vi "Set Attenuation, 400 MHz Power, and 2.45 GHz Power.vi"(6 "2.45 GHz Wake-Up Power (6)":i8(ring)=6 items=["-29"=-29, "-4"=-4, "-2"=-2, "0"=0, "2"=2, "4"=4, "6"=6, "8"=8, "10"=10, "12"=12, "14"=14, "16"=16, "18"=18, "20"=20, "22"=22, "24"=24, "26"=26, "27"=27], 8 "error in":errorcluster, 9 "Attenuation dB (0)":dbl, 10 "400 MHz MICS Power Setting (0x16)":u8=22 format="%.0x", 11 "VISA Resource Name":refnum<visa-resource-name>) -> (0 "error out":errorcluster, 3 "dup VISA Resource Name":refnum<visa-resource-name>)   [LabVIEW 2020]
uses:
  MICS Parameters Global.vi
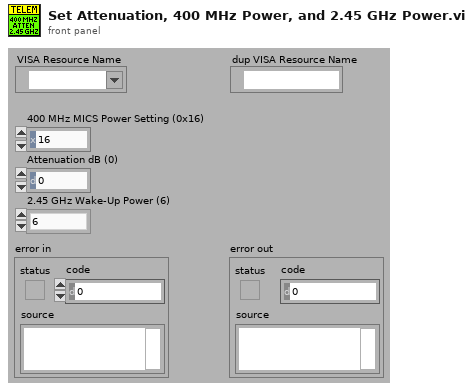
[diagram p1: front panel]
types:
  T1 = cluster{"ConfigFlags":u8, "ImplantID":u32, "CompanyID":u8, "Normal_Comm":cluster{"RF_Channel":u8, "UserData":u8, "TX_Mod":u8, "RX_Mod":u8, "RX_BlockSize":u8, "BlockPerPack":u8, "TX_BlockSize":u8}, "Emerg_Comm":cluster{"RF_Channel":u8, "UserData":u8, "TX_Mod":u8, "RX_Mod":u8, "TX_BlockSize":u8, "BlockPerPack":u8, "RX_BlockSize":u8}, "ImplantRev":u8, "245TX_PowerCal":i8, "245TX_Power":i8, "CCA_RSSI_Thresholds":cluster{"ch0":u16, "ch1":u16, "ch2":u16, "ch3":u16, "ch4":u16, "ch5":u16, "ch6":u16, "ch7":u16, "ch8":u16, "ch9":u16}}
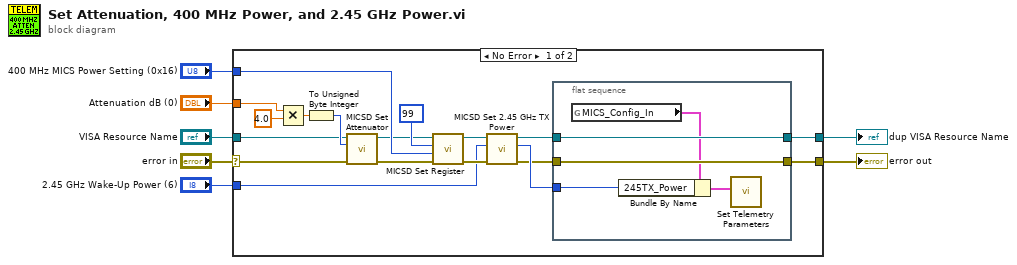
[diagram p0: block diagram]
diagram:
  n1 = case shown="No Error" "error in" {
    selector: "error in" -> [w12 w31]
    tunnel: "400 MHz MICS Power Setting (0x16)" -> [w25 _]
    tunnel: "Attenuation dB (0)" -> [w20 _]
    tunnel: "VISA Resource Name" -> [w17 w32]
    tunnel: [w10 w32] -> w4
    tunnel: [w8 w31] -> w3
    tunnel: "2.45 GHz Wake-Up Power (6)" -> [w13 _]
    frame No Error {
      n2 = Multiply(x=w20, y=4.0) -> (x*y=w18:dbl)
      n3 = To Unsigned Byte Integer(number=w18) -> (unsigned 8bit integer=w21:u8)
      n4 = call "MICSD Set Attenuator.vi"("error in (no error)"=w12, "Attenuation"=w21, "VISA Resource Name"=w17) -> ("error out"=w23:errorcluster, "dup VISA Resource Name"=w22:refnum<visa-resource-name>)  [unwired: 7 in]
      n5 = call "MICSD Set Register.vi"("error in (no error)"=w23, "Data"=w25, "Address"=u16 99, "VISA Resource Name"=w22) -> ("error out"=w15:errorcluster, "dup VISA Resource Name"=w16:refnum<visa-resource-name>)  [unwired: 6 in]
      n6 = call "MICSD Set 2.45 GHz TX Power.vi"("error in (no error)"=w15, "245TX_Power"=w13, "VISA Resource Name"=w16) -> ("error out"=w9:errorcluster, "dup 245TX_Power"=w14:i8, "dup VISA Resource Name"=w11:refnum<visa-resource-name>)  [unwired: 6 in]
      n7 = flat-sequence {
        tunnel: w14 -> [w30]
        tunnel: w11 -> [w28]
        tunnel: [w28] -> w10
        tunnel: w9 -> [w27]
        tunnel: [w27] -> w8
        frame #0 {
          n8 = global read "MICS Parameters Global.vi" "MICS_Config_In"() -> (w26:T1)
          n9 = Bundle By Name(cluster=w26, "245TX_Power"=w30) -> (w29:T1)
          n10 = call "Set Telemetry Parameters.vi"("MICS_Config_In"=w29) -> ()  [unwired: 11 in]
        }
      }
    }
    frame Error {
    }
  }
  "error out" <- w3
  "dup VISA Resource Name" <- w4
